vi "obtain_image_pixels.vi"(8 "error in (no error)":errorcluster, 10 "index":i32, 11 "ImageCollection in":refnum<class "ImageCollection.lvclass">=refnum) -> (0 "error out":errorcluster, 2 "Image Pixels (Float)":sgl[][](array[numeric]) format="%.2f", 3 "ImageCollection out":refnum<class "ImageCollection.lvclass">)   [LabVIEW 2010]
uses:
  bricks/classes/ImageCollection/ImageCollection.lvclass
  bricks/classes/Image/Image.lvclass
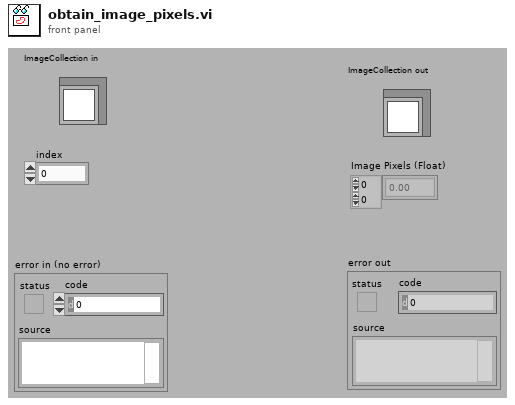
[diagram p1: front panel]
types:
  T1 = typedef "IMAQ Image.ctl" = refnum<image>
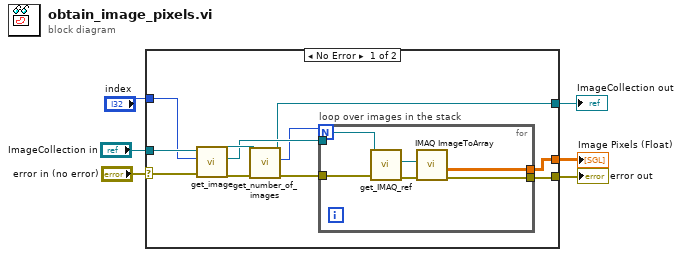
[diagram p0: block diagram]
diagram:
  n1 = case shown="No Error" "error in (no error)" {
    selector: "error in (no error)" -> [w12 w25]
    tunnel: "ImageCollection in" -> [w17 w24]
    tunnel: [w10 _] -> w5
    tunnel: [w11 w25] -> w3
    tunnel: [w9 w24] -> w2
    tunnel: "index" -> [w8 _]
    frame No Error {
      n2 = call-dynamic "get_image.vi"("error in (no error)"=w12, "index"=w8, "ImageCollection in"=w17) -> ("error out"=w15:errorcluster, "Image.lvclass"=w14:refnum<class "Image.lvclass">, "ImageCollection out"=w16:refnum<class "ImageCollection.lvclass">)  [unwired: 6 in]
      n3 = call-dynamic "get_number_of_images.vi"("error in (no error)"=w15, "ImageCollection in"=w16) -> ("error out"=w13:errorcluster, "size"=w7:i32, "ImageCollection out"=w9:refnum<class "ImageCollection.lvclass">)  [unwired: 7 in]
      n4 = for "loop over images in the stack" {
        N: w7 -> [_]
        tunnel: w14 -> [w23]
        tunnel: w13 -> [w22]
        tunnel: [w19] -> w11
        tunnel: [w18] -> w10
        n5 = call-dynamic "get_IMAQ_ref.vi"("error in (no error)"=w22, "Image.lvclass in"=w23) -> ("error out"=w20:errorcluster, "Image"=w21:T1)  [unwired: 5 in, 3 out]
        n6 = call "IMAQ ImageToArray"("error in (no error)"=w20, "Image"=w21) -> ("Image Pixels (Float)"=w18:sgl[][], "error out"=w19:errorcluster)  [unwired: 2 in, 3 out]
      }
    }
    frame Error {
    }
  }
  "Image Pixels (Float)" <- w5
  "error out" <- w3
  "ImageCollection out" <- w2
